vi "Create Plugin Groups.vi"(8 "error in (no error)":errorcluster, 9 "String":string, 10 "dsf refnum in":refnum<class "Configuration Session.lvclass">, 11 "Section Ptr":T1 format="%.0x") -> (0 "error out":errorcluster)   [LabVIEW 2017, in "Data Sharing Framework System Explorer.lvlib"]
uses:
  Data Sharing Framework System Explorer.lvlib
  <vilib>/NI Veristand/Custom Device API/Custom Device Item Ref.ctl
  Engine/DSF Core.lvlibp/Classes/Configuration/Configuration Session.lvclass
  Engine/DSF Core.lvlibp/Classes/Configuration/Read Plugin Group IDs.vi
  Engine/DSF Core.lvlibp/Classes/Configuration/Read Group.vi
  <vilib>/NI Veristand/Custom Device API/Custom Device API.lvlib
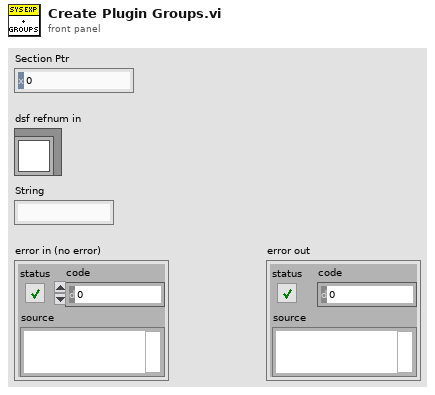
[diagram p1: front panel]
types:
  T1 = typedef "Custom Device API.lvlib/Custom Device Item Ref.ctl" = u64
  T2 = typedef "DSF Core.lvlibp/DSF Group Info.ctl" = cluster{"direction":T3, "timing":T4, "transfer ids":string[], "settings id":string, "thread":i32, "timeout behavior":T5}
  T3 = typedef "DSF Core.lvlibp/DSF Direction.ctl" = enum8{"Tx", "Rx"}
  T4 = typedef "DSF Core.lvlibp/DSF Timing Info.ctl" = cluster{"priority":u64, "decimation":u64, "offset":u64}
  T5 = typedef "DSF Core.lvlibp/DSF Timeout Behavior.ctl" = enum8{"Increment Late Count", "Throw Error"}
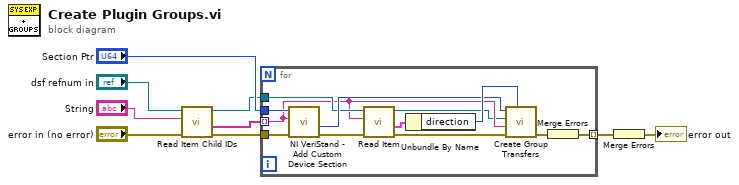
[diagram p0: block diagram]
diagram:
  n1 = call-poly "Read Item Child IDs.vi"("error in (no error)"="error in (no error)", "Plugin ID"="String", "Configuration Session"="dsf refnum in") -> ("error out"=w4:errorcluster, "Group IDs"=w3:string[], "Configuration Session out"=w2:refnum<class "Configuration Session.lvclass">)  [unwired: 5 in, 1 out]
  n2 = for {
    tunnel: w3 -> [w13] mode=indexing
    tunnel: "Section Ptr" -> [w21]
    tunnel: w4 -> [w20]
    tunnel: [w19] -> w8 mode=indexing
    tunnel: w2 -> [w15]
    n3 = call <vilib>:"NI VeriStand - Add Custom Device Section.vi"("error in (no error)"=w20, "Section Name"=w13, "Parent Ref in"=w21) -> ("error out"=w14:errorcluster, "Section Ptr"=w16:T1)  [unwired: 5 in, 2 out]
    n4 = call-poly "Read Item.vi"("error in (no error)"=w14, "Group ID"=w13, "Configuration Session in"=w15) -> ("error out"=w11:errorcluster, "value"=w10:T2, "Configuration Session out"=w12:refnum<class "Configuration Session.lvclass">)  [unwired: 5 in, 1 out]
    n5 = Unbundle By Name(w10) -> ("direction"=w18:T3)
    n6 = call "Create Group Transfers.vi"("direction"=w18, "error in (no error)"=w11, "Group ID"=w13, "dsf refnum in"=w12, "Section Ptr"=w16) -> ("error out"=w17:errorcluster)  [unwired: 6 in]
    n7 = Merge Errors(w17) -> (w19:errorcluster)
  }
  n8 = Merge Errors(w8) -> (→"error out":errorcluster)
